vi "Register New Object.vi"(6 "timeout (100 ms)":i32, 10 "New Object Name":string, 11 "Owner Fully Qualified Name":string) -> (0 "timed out":bool, 1 "operation complete":bool, 3 "New UniqueName Object":refnum<class "UniqueName.lvclass">)   [LabVIEW 2014, in "UniqueName.lvlib" / "UniqueName.lvclass"]
uses:
  UniqueName.lvclass
  Command.ctl
  UniqueName.lvclass/UniqueName.ctl
  UniquenessCriteria/UniquenessCriteria.lvclass/UniquenessCriteria.ctl
  Key.ctl
  Write UUID.vi
  RandomStringGenerator/Generate Random String.vi
  UniquenessCriteria/UniquenessCriteria.lvclass
  NameIncrementAlgorithm/StringIncrementAlgorithm.lvclass
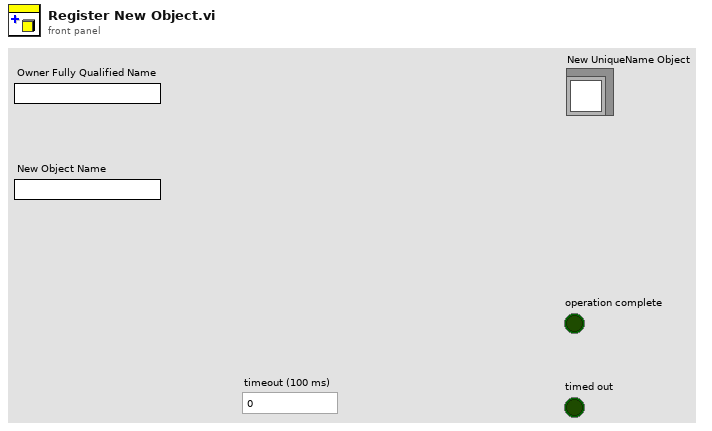
[diagram p1: front panel]
types:
  T1 = typedef "UniqueName.lvlib/UniqueName.lvclass/Command.ctl" = enum16{"Get", "Get All", "Set", "Delete", "Get Status", "Init", "Reserve Ownership", "Release Ownership", "Lock", "Unlock"}
  T2 = typedef "UniqueName.lvlib/UniqueName.lvclass/RegistryStatus.ctl" = cluster{"Registry Configuration":T3, "Registry Owned":bool, "Write-Protected":bool, "Owned":bool, "Released":bool, "Locked":bool, "Unlocked":bool}
  T3 = typedef "UniqueName.lvlib/UniqueName.lvclass/RegistryConfiguration.ctl" = cluster{"Delimiter":refnum<class "Delimiter.lvclass">, "RandomStringGenerator":refnum<class "RandomStringGenerator.lvclass">, "UniquenessCriteria":refnum<class "UniquenessCriteria.lvclass">, "StringIncrement":refnum<class "StringIncrementAlgorithm.lvclass">}
  T4 = typedef "UniqueName.lvlib/UniqueName.lvclass/Key.ctl" = enum16{"Fully Qualified Name", "Unique Name", "Given Name", "Parent Fully Qualified Name"}
  T5 = typedef "UniqueName.lvlib/UniquenessCriteria.lvclass/Criteria.ctl" = enum16{"Globally-Unique Fully Qualified Name", "Globally-Unique Name"}
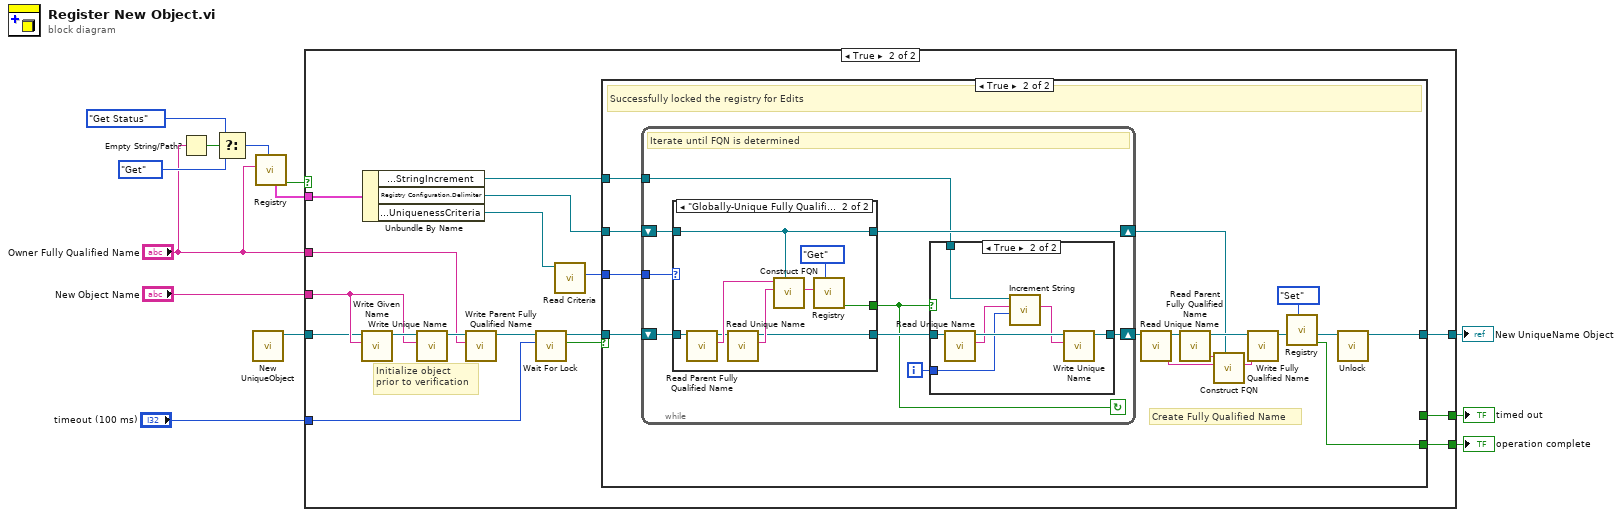
[diagram p0: block diagram]
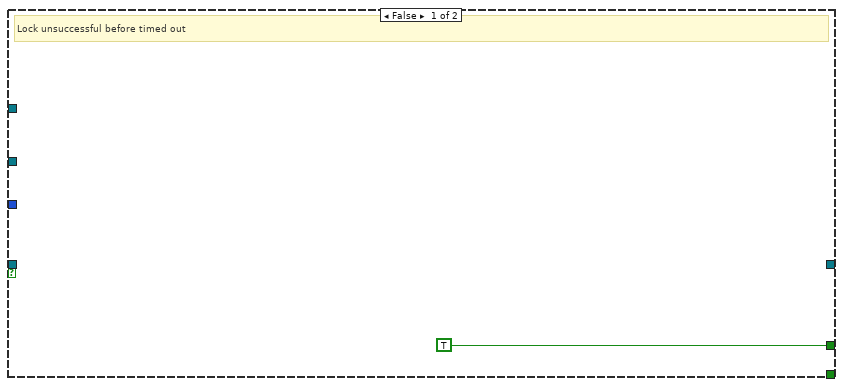
[diagram p3: hidden frame]
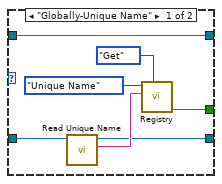
[diagram p5: hidden frame]
diagram:
  n1 = Empty String/Path?(string/path="Owner Fully Qualified Name") -> (empty?=w7:bool)
  n2 = Select(t=Command."Get Status" ("Command (Get)"), s=w7, f=Command."Get" ("Command (Get)")) -> (s? t:f=w4:T1)
  n3 = call "New UniqueObject.vi"() -> ("UniqueName out"=w8:refnum<class "UniqueName.lvclass">)  [unwired: 11 in]
  n4 = call "Registry.vi"("Command (Get)"=w4, "Search term (Get & Delete Operations)"="Owner Fully Qualified Name") -> ("Found or Completed?"=w2:bool, "Registry Status"=w10:T2)  [unwired: 5 in, 3 out]
  n5 = case shown="True" w2 {
    tunnel: "New Object Name" -> [_ w28]
    tunnel: [_ w27] -> w12
    tunnel: [_ w25] -> w11
    tunnel: w10 -> [_ w24]
    tunnel: "timeout (100 ms)" -> [_ w22]
    tunnel: w8 -> [_ w17]
    tunnel: "Owner Fully Qualified Name" -> [_ w15]
    tunnel: [_ w14] -> w1
    frame False {
    }
    frame True {
      # "Initialize object\nprior to verification"
      n6 = call "Write Given Name.vi"("Given Name"=w28, "UniqueName in"=w17) -> ("UniqueName out"=w30:refnum<class "UniqueName.lvclass">)  [unwired: 9 in]
      n7 = Unbundle By Name(w24) -> ("Registry Configuration.StringIncrement"=w19:refnum<class "StringIncrementAlgorithm.lvclass">, "Registry Configuration.Delimiter"=w20:refnum<class "Delimiter.lvclass">, "Registry Configuration.UniquenessCriteria"=w21:refnum<class "UniquenessCriteria.lvclass">)
      n8 = call "Write Unique Name.vi"("Unique Name"=w28, "UniqueName in"=w30) -> ("UniqueName out"=w29:refnum<class "UniqueName.lvclass">)  [unwired: 9 in]
      n9 = call "Write Parent Fully Qualified Name.vi"("Parent Fully Qualified Name"=w15, "UniqueName in"=w29) -> ("UniqueName out"=w16:refnum<class "UniqueName.lvclass">)  [unwired: 9 in]
      n10 = call "Wait For Lock.vi"("timeout (100 ms)"=w22, "UniqueName in"=w16) -> ("Locked"=w26:bool, "UniqueName out"=w18:refnum<class "UniqueName.lvclass">)  [unwired: 8 in]
      n11 = call "Read Criteria.vi"("UniquenessCriteria in"=w21) -> ("Criteria"=w23:T5)  [unwired: 9 in, 1 out]
      n12 = case shown="True" w26 {
        tunnel: w23 -> [_ w46]
        tunnel: w18 -> [_ w39]
        tunnel: [_ w36] -> w27
        tunnel: [TRUE _] -> w25
        tunnel: w20 -> [_ w35]
        tunnel: w19 -> [_ w34]
        tunnel: [_ w32] -> w14
        frame False {
          # "Lock unsuccessful before timed out"
        }
        frame True {
          # "Create Fully Qualified Name"
          # "Successfully locked the registry for Edits"
          n13 = while {
            tunnel: w46 -> [w56]
            shift-right: [w54] -> w42
            shift-left: w39 -> [w53]
            shift-right: [w50] -> w38
            shift-left: w35 -> [w51]
            tunnel: w34 -> [w49]
            i -> [w48]
            stop <- w52 continue-if-true
            # "Iterate until FQN is determined"
            n14 = case shown="\"Globally-Unique Fully Qualified Name\"" w56 {
              tunnel: [w69 w79] -> w52
              tunnel: w53 -> [w68 w74]
              tunnel: [w66 w72] -> w55
              tunnel: w51 -> [w65 w75]
              tunnel: [w65 w75] -> w50
              frame "Globally-Unique Name" {
                n15 = call "Read Unique Name.vi"("UniqueName in"=w68) -> ("Unique Name"=w67:string, "UniqueName out"=w66:refnum<class "UniqueName.lvclass">)  [unwired: 9 in]
                n16 = call "Registry.vi"("Command (Get)"=Command."Get", "Search term (Get & Delete Operations)"=w67, "Key (FQN)"=Key."Unique Name") -> ("Found or Completed?"=w69:bool)  [unwired: 4 in, 4 out]
              }
              frame "Globally-Unique Fully Qualified Name" {
                n17 = call "Read Parent Fully Qualified Name.vi"("UniqueName in"=w74) -> ("Parent Fully Qualified Name"=w77:string, "UniqueName out"=w73:refnum<class "UniqueName.lvclass">)  [unwired: 9 in]
                n18 = call "Read Unique Name.vi"("UniqueName in"=w73) -> ("Unique Name"=w76:string, "UniqueName out"=w72:refnum<class "UniqueName.lvclass">)  [unwired: 9 in]
                n19 = call "Construct FQN.vi"("Delimiter"=w75, "Name"=w76, "Parent FQN"=w77) -> ("FQN"=w78:string)  [unwired: 8 in]
                n20 = call "Registry.vi"("Command (Get)"=Command."Get", "Search term (Get & Delete Operations)"=w78) -> ("Found or Completed?"=w79:bool)  [unwired: 5 in, 4 out]
              }
            }
            n21 = case shown="True" w52 {
              tunnel: w55 -> [w57 w63]
              tunnel: [w57 w64] -> w54
              tunnel: w49 -> [_ w61]
              tunnel: w48 -> [_ w58]
              frame False {
                # "Name already unique"
              }
              frame True {
                n22 = call "Read Unique Name.vi"("UniqueName in"=w63) -> ("Unique Name"=w60:string, "UniqueName out"=w62:refnum<class "UniqueName.lvclass">)  [unwired: 9 in]
                n23 = call "Increment String.vi"("Numeric"=w58, "Input String"=w60, "String Increment Algorithm"=w61) -> ("Incremented String"=w59:string)  [unwired: 8 in]
                n24 = call "Write Unique Name.vi"("Unique Name"=w59, "UniqueName in"=w62) -> ("UniqueName out"=w64:refnum<class "UniqueName.lvclass">)  [unwired: 9 in]
              }
            }
          }
          n25 = call "Read Unique Name.vi"("UniqueName in"=w42) -> ("Unique Name"=w40:string, "UniqueName out"=w43:refnum<class "UniqueName.lvclass">)  [unwired: 9 in]
          n26 = call "Read Parent Fully Qualified Name.vi"("UniqueName in"=w43) -> ("Parent Fully Qualified Name"=w45:string, "UniqueName out"=w44:refnum<class "UniqueName.lvclass">)  [unwired: 9 in]
          n27 = call "Construct FQN.vi"("Delimiter"=w38, "Name"=w40, "Parent FQN"=w45) -> ("FQN"=w41:string)  [unwired: 8 in]
          n28 = call "Write Fully Qualified Name.vi"("Fully Qualified Name"=w41, "UniqueName in"=w44) -> ("UniqueName out"=w33:refnum<class "UniqueName.lvclass">)  [unwired: 9 in]
          n29 = call "Registry.vi"("Command (Get)"=Command."Set", "UniqueName Object (Set)"=w33) -> ("Found or Completed?"=w32:bool, "Returned Object"=w37:refnum<class "UniqueName.lvclass">)  [unwired: 5 in, 3 out]
          n30 = call "Unlock.vi"("UniqueName in"=w37) -> ("UniqueName out"=w36:refnum<class "UniqueName.lvclass">)  [unwired: 10 in]
        }
      }
    }
  }
  "New UniqueName Object" <- w12
  "timed out" <- w11
  "operation complete" <- w1
